vi "Write Base URL.vi"(8 "error in (no error)":errorcluster, 10 "Base URL":string, 11 "REST Client in":refnum<class "REST Client.lvclass">) -> (0 "error out":errorcluster, 3 "REST Client out":refnum<class "REST Client.lvclass">)   [LabVIEW 2013, in "REST Client.lvlib" / "REST Client.lvclass"]
doc: "Write Base URL"
uses:
  REST Client.lvclass
  REST Client.lvclass/REST Client.ctl
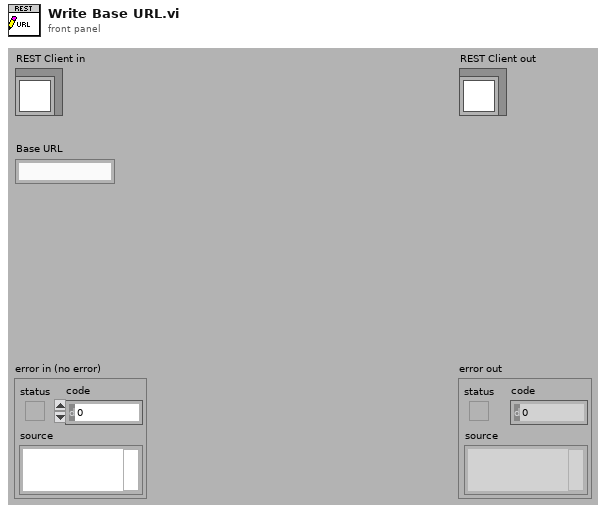
[diagram p1: front panel]
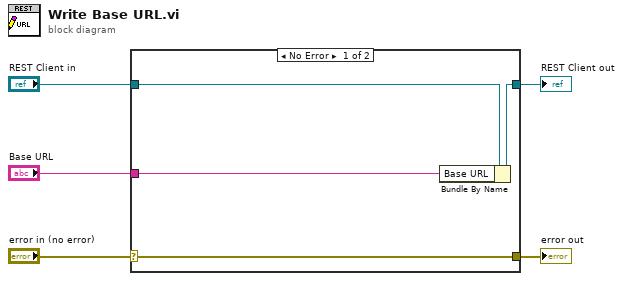
[diagram p0: block diagram]
diagram:
  n1 = case shown="No Error" "error in (no error)" {
    selector: "error in (no error)" -> [w9 w10]
    tunnel: [w9 w10] -> w4
    tunnel: [w7 w11] -> w2
    tunnel: "REST Client in" -> [w8 w11]
    tunnel: "Base URL" -> [w6 _]
    frame No Error {
      n2 = Bundle By Name(cluster=w8, "Base URL"=w6) -> (w7:refnum<class "REST Client.lvclass">)
    }
    frame Error {
    }
  }
  "error out" <- w4
  "REST Client out" <- w2
